vi "Pre-Install Custom Action.vi"(10 "Variant":variant) -> (0 "error out":errorcluster)   [LabVIEW 2020]
uses:
  <resource>/dialog/lvconfig.llb/LV Config Read String.vi
  <resource>/dialog/lvconfig.llb/LV Config Read Numeric (I32).vi
  <vilib>/Utility/config.llb/Write Key (String).vi
  <vilib>/Utility/config.llb/Write Key (I32).vi
  <vilib>/Utility/config.llb/NI_LVConfig.lvlib
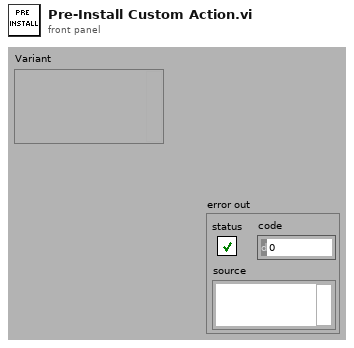
[diagram p1: front panel]
types:
  T1 = typedef "NI_LVConfig.lvlib/Config Data RefNum.ctl" = refnum<k1>
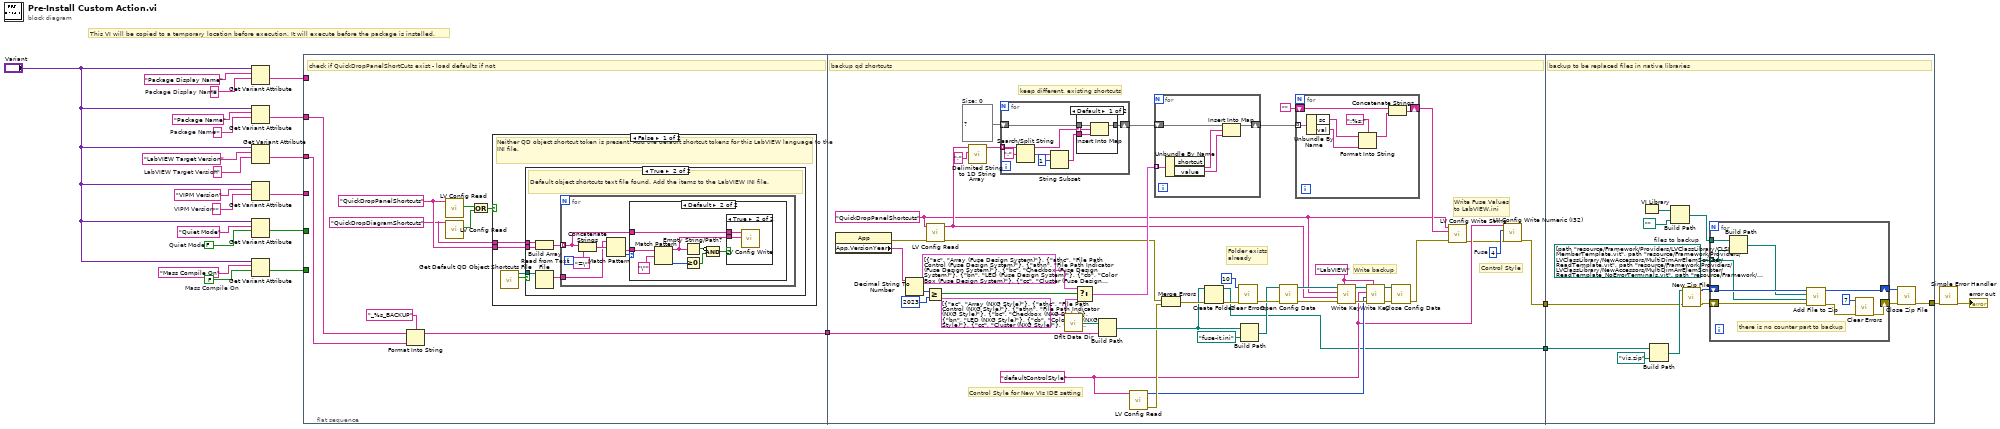
[diagram p0: block diagram]
diagram:
  w6 = FALSE  # Mass Compile On
  w8 = ""  # Package Display Name
  w15 = FALSE  # Quiet Mode
  w18 = ""  # VIPM Version
  w20 = ""  # LabVIEW Target Version
  w22 = ""  # Package Name
  # "This VI will be copied to a temporary location before execution. It will execute before the package is installed."
  n1 = Get Variant Attribute(Variant="Variant", name="Package Display Name", default value (empty Variant)=w8) -> (value=w14:string)  [unwired: 1 in, 3 out]
  n2 = Get Variant Attribute(Variant="Variant", name="Package Name", default value (empty Variant)=w22) -> (value=w13:string)  [unwired: 1 in, 3 out]
  n3 = Get Variant Attribute(Variant="Variant", name="LabVIEW Target Version", default value (empty Variant)=w20) -> (value=w12:string)  [unwired: 1 in, 3 out]
  n4 = Get Variant Attribute(Variant="Variant", name="VIPM Version", default value (empty Variant)=w18) -> (value=w11:string)  [unwired: 1 in, 3 out]
  n5 = Get Variant Attribute(Variant="Variant", name="Quiet Mode", default value (empty Variant)=w15) -> (value=w10:bool)  [unwired: 1 in, 3 out]
  n6 = Get Variant Attribute(Variant="Variant", name="Mass Compile On", default value (empty Variant)=w6) -> (value=w9:bool)  [unwired: 1 in, 3 out]
  n7 = flat-sequence {
    tunnel: w14 -> [_]
    tunnel: w13 -> [w27]
    tunnel: w12 -> [w26]
    tunnel: w11 -> [_]
    tunnel: w10 -> [_]
    tunnel: w9 -> [_]
    tunnel: [w25] -> w4
    tunnel: w4 -> [w85]
    tunnel: [w59] -> w3
    tunnel: [w64] -> w2
    tunnel: [w129] -> w5
    tunnel: w3 -> [w126]
    tunnel: w2 -> [w128]
    frame #0 {
      w32 = "QuickDropDiagramShortcuts" ("Name")
      w33 = "QuickDropPanelShortcuts" ("key")
      # "check if QuickDropPanelShortCuts exist - load defaults if not"
      n8 = Format Into String(format string="_%s_BACKUP", initial string=w27, w26) -> (resulting string=w25:string)  [unwired: 1 in, 1 out]
      n9 = call-poly <resource>:"LV Config Read.vi"("key"=w33) -> ("found?"=w29:bool)  [unwired: 4 in, 2 out]
      n10 = call-poly <resource>:"LV Config Read.vi"("key"=w32) -> ("found?"=w30:bool)  [unwired: 4 in, 2 out]
      n11 = Or(x=w29, y=w30) -> (x .or. y?=w31:bool)
      n12 = case shown="False" w31 {
        tunnel: w32 -> [w37 _]
        tunnel: w33 -> [w36 _]
        frame False {
          # "Neither QD object shortcut token is present. Add the default shortcut tokens for this LabVIEW language to the INI file."
          n13 = call <resource>:"Get Default QD Object Shortcuts File.vi"() -> ("file exists"=w35:bool, "default shortcuts text file"=w34:path)  [unwired: 10 in]
          n14 = case shown="True" w35 {
            tunnel: w34 -> [_ w42]
            tunnel: w37 -> [_ w40]
            tunnel: w36 -> [_ w39]
            frame False {
              # "Default object shortcuts text file does not exist for this language. Do nothing."
            }
            frame True {
              # "Default object shortcuts text file found. Add the items to the LabVIEW INI file."
              n15 = Build Array(w40, w39) -> (w38:string[])
              n16 = Read from Text File(file (use dialog)=w42) -> (text=w41:string)  [unwired: 3 in, 3 out]
              n17 = for {
                tunnel: w41 -> [w44]
                tunnel: w38 -> [w46] mode=indexing
                n18 = Concatenate Strings(w46, "=\"") -> (w45:string)
                n19 = Match Pattern(string=w44, regular expression=w45) -> (after substring=w47:string, offset past match=w43:i32)  [unwired: 1 in, 2 out]
                n20 = case shown="Default" w43 {
                  tunnel: w47 -> [_ w56]
                  tunnel: w46 -> [_ w54]
                  frame -1 {
                  }
                  frame Default {
                    n21 = Match Pattern(string=w56, regular expression="\"") -> (before substring=w53:string, offset past match=w51:i32)  [unwired: 1 in, 2 out]
                    n22 = Empty String/Path?(string/path=w53) -> (empty?=w52:bool)
                    n23 = Greater Or Equal To 0?(x=w51) -> (x >= 0?=w50:bool)
                    n24 = Compound Arithmetic op=AND(invert w52, w50) -> (w49:bool)
                    n25 = case shown="True" w49 {
                      tunnel: w54 -> [_ w58]
                      tunnel: w53 -> [_ w57]
                      frame False {
                      }
                      frame True {
                        n26 = call-poly <resource>:"LV Config Write.vi"("value"=w57, "key"=w58) -> ()  [unwired: 5 in, 1 out]
                      }
                    }
                  }
                }
              }
            }
          }
        }
        frame True {
          # "One or both of the QD object shortcut tokens is already present, don't do anything with loading default shortcuts."
        }
      }
    }
    frame #1 {
      w62 = u32 4  # Fuse
      w63 = "defaultControlStyle" ("key")
      w98 = map{string, string} {}  # Size: 0
      w60 = "QuickDropPanelShortcuts" ("key")
      w72 = "LabVIEW" ("section")
      # "Write backup"
      # "Write Fuse Values\nto LabVIEW.ini"
      # "keep different, existing shortcuts"
      # "Control Style"
      # "Control Style for New VIs IDE setting"
      # "Folder exists\nalready"
      # "backup qd shortcuts"
      n27 = property class="App"() -> (error out=w71:errorcluster, "App.VersionYear"=w91:string)  [unwired: 2 in, 1 out]
      n28 = Decimal String To Number(string=w91) -> (number=w90:i32)  [unwired: 2 in, 1 out]
      n29 = Greater Or Equal?(x=w90, y=2023) -> (x >= y?=w88:bool)
      n30 = call-poly <resource>:"LV Config Read.vi"("error in"=w71, "key"=w60) -> ("error out"=w70:errorcluster, "value"=w69:string)  [unwired: 3 in, 1 out]
      n31 = call <vilib>:"Delimited String to 1D String Array.vi"("delimiter"=";", "delimited string"=w69) -> ("string array"=w99:string[])  [unwired: 9 in]
      n32 = for {
        tunnel: w99 -> [w119] mode=indexing
        shift-right: [w117] -> w97
        shift-left: w98 -> [w118]
        n33 = Search/Split String(string=w119, search string/char (-)=":") -> (substring before match=w116:string, match + rest of string=w115:string)  [unwired: 1 in, 1 out]
        n34 = String Subset(string=w115, offset (0)=1) -> (substring=w114:string)  [unwired: 1 in]
        n35 = case shown="Default" w116 {
          selector: w116 -> [w122 _]
          tunnel: w118 -> [w124 w125]
          tunnel: [w123 w125] -> w117
          tunnel: w114 -> [w121 _]
          frame Default {
            n36 = Insert Into Map(map in=w124, key=w122, value=w121) -> (map out=w123:map{string, string})  [unwired: 2 out]
          }
          frame "" {
          }
        }
      }
      n37 = call <vilib>:"Dflt Data Dir.vi"() -> ("App:Default Data Directory"=w87:path)
      n38 = Select(t=cluster{"shortcut":string, "value":string}[] [{"shortcut"="ac", "value"="Array (Fuse Design System)"}, {"shortcut"="athc", "value"="File Path Control (Fuse Design System)"}, {"shortcut"="athn", "value"="File Path Indicator (Fuse Design System)"}, {"shortcut"="bc", "value"="Checkbox (Fuse Design System)"}, {"shortcut"="bn", "value"="LED (Fuse Design System)"}, {"shortcut"="cb", "value"="Color Box (Fuse Design System)"}, {"shortcut"="cc", "value"="Cluster (Fuse Design System)"}, {"shortcut"="cr", "value"="Control Refnum"}, {"shortcut"="en", "value"="Enum (Fuse Design System)"}, {"shortcut"="erc", "value"="Error In  (Fuse Design System)"}, {"shortcut"="ern", "value"="Error Out (Fuse Design System)"}, {"shortcut"="nc", "value"="Numeric Control (Fuse Design System)"}, {"shortcut"="nn", "value"="Numeric Indicator (Fuse Design System)"}, {"shortcut"="sac", "value"="Select a Control..."}, {"shortcut"="sc", "value"="String Control (Fuse Design System)"}, {"shortcut"="sn", "value"="String Indicator (Fuse Design System)"}, {"shortcut"="vr", "value"="VI Refnum"}, {"shortcut"="wc", "value"="Waveform Chart (Fuse Design System)"}, {"shortcut"="wg", "value"="Waveform Graph (Fuse Design System)"}, {"shortcut"="xg", "value"="XY Graph (Fuse Design System)"}] ("Array"), s=w88, f=cluster{"shortcut":string, "value":string}[] [{"shortcut"="ac", "value"="Array (NXG Style)"}, {"shortcut"="athc", "value"="File Path Control (NXG Style)"}, {"shortcut"="athn", "value"="File Path Indicator (NXG Style)"}, {"shortcut"="bc", "value"="Checkbox (NXG Style)"}, {"shortcut"="bn", "value"="LED (NXG Style)"}, {"shortcut"="cb", "value"="Color Box (NXG Style)"}, {"shortcut"="cc", "value"="Cluster (NXG Style)"}, {"shortcut"="cr", "value"="Control Refnum"}, {"shortcut"="en", "value"="Enum (NXG Style)"}, {"shortcut"="erc", "value"="Error In  (NXG Style)"}, {"shortcut"="ern", "value"="Error Out (NXG Style)"}, {"shortcut"="nc", "value"="Numeric Control (NXG Style)"}, {"shortcut"="nn", "value"="Numeric Indicator (NXG Style)"}, {"shortcut"="sac", "value"="Select a Control..."}, {"shortcut"="sc", "value"="String Control (NXG Style)"}, {"shortcut"="sn", "value"="String Indicator (NXG Style)"}, {"shortcut"="vr", "value"="VI Refnum"}, {"shortcut"="wc", "value"="Waveform Chart (NXG Style)"}, {"shortcut"="wg", "value"="Waveform Graph (NXG Style)"}, {"shortcut"="xg", "value"="XY Graph (NXG Style)"}] ("Array")) -> (s? t:f=w93:cluster{"shortcut":string, "value":string}[])
      n39 = Build Path(base path=w87, name or relative path=w85) -> (appended path=w73:path)
      n40 = call-poly <resource>:"LV Config Read.vi"("key"=w63) -> ("error out"=w68:errorcluster, "value"=w67:i32)  [unwired: 4 in, 1 out]
      n41 = for {
        tunnel: w93 -> [w110] mode=indexing
        shift-right: [w111] -> w96
        shift-left: w97 -> [w112]
        n42 = Unbundle By Name(w110) -> ("shortcut"=w109:string, "value"=w108:string)
        n43 = Insert Into Map(map in=w112, key=w109, value=w108) -> (map out=w111:map{string, string})  [unwired: 2 out]
      }
      n44 = Merge Errors(w70, w68) -> (w74:errorcluster)
      n45 = Create Folder(path (use dialog)=w73, error in=w74) -> (created path=w59:path, error out=w75:errorcluster)  [unwired: 1 in, 1 out]
      n46 = call <vilib>:"Clear Errors.vi"("error in (no error)"=w75, "specific error code to clear (0: all)"=10) -> ("error out"=w84:errorcluster)  [unwired: 4 in, 1 out]
      n47 = Build Path(base path=w73, name or relative path=path "fuse-it.ini") -> (appended path=w76:path)
      n48 = call <vilib>:"Open Config Data.vi"("error in (no error)"=w84, "configuration file path"=w76) -> ("error out"=w82:errorcluster, "refnum"=w81:T1)  [unwired: 7 in, 1 out]
      n49 = for {
        tunnel: w96 -> [w107] mode=indexing
        shift-right: [w103] -> w65
        shift-left: "" -> [w105]
        n50 = Unbundle By Name(w107) -> ("sc"=w101:string, "val"=w102:string)
        n51 = Format Into String(format string=":%s;", initial string=w101, w102) -> (resulting string=w104:string)  [unwired: 1 in, 1 out]
        n52 = Concatenate Strings(w105, w104) -> (w103:string)
      }
      n53 = call-poly <vilib>:"Write Key.vi"("section"=w72, "error in (no error)"=w82, "value"=w69, "key"=w60, "refnum"=w81) -> ("error out"=w80:errorcluster, "refnum out"=w79:T1)  [unwired: 4 in, 1 out]
      n54 = call-poly <vilib>:"Write Key.vi"("section"=w72, "error in (no error)"=w80, "value"=w67, "key"=w63, "refnum"=w79) -> ("error out"=w78:errorcluster, "refnum out"=w77:T1)  [unwired: 4 in, 1 out]
      n55 = call <vilib>:"Close Config Data.vi"("error in (no error)"=w78, "refnum"=w77) -> ("error out"=w66:errorcluster)  [unwired: 8 in, 1 out]
      n56 = call <resource>:"LV Config Write String.vi"("error in (no error)"=w66, "value"=w65, "key"=w60) -> ("error out"=w61:errorcluster)  [unwired: 4 in]
      n57 = call <resource>:"LV Config Write Numeric (I32).vi"("error in (no error)"=w61, "value"=w62, "key"=w63) -> ("error out"=w64:errorcluster)  [unwired: 4 in]
    }
    frame #2 {
      w127 = path[] [path "resource/Framework/Providers/LVClassLibrary/CLSUIP_MemberTemplate.vit", path "resource/Framework/Providers/LVClassLibrary/NewAccessors/MultiDimArrElemScripter/ReadTemplate.vit", path "resource/Framework/Providers/LVClassLibrary/NewAccessors/MultiDimArrElemScripter/ReadTemplate_NoErrorTerminals.vit", path "resource/Framework/Providers/LVClassLibrary/NewAccessors/MultiDimArrElemScripter/WriteTemplate.vit", path "resource/Framework/Providers/LVClassLibrary/NewAccessors/MultiDimArrElemScripter/WriteTemplate_NoErrorTerminals.vit", path "resource/Framework/Providers/LVClassLibrary/NewAccessors/BaseAccessorScripter/ReadTemplate.vit", path "resource/Framework/Providers/LVClassLibrary/NewAccessors/BaseAccessorScripter/ReadTemplate_NoErrorTerminals.vit", path "resource/Framework/Providers/LVClassLibrary/NewAccessors/BaseAccessorScripter/WriteTemplate.vit", path "resource/Framework/Providers/LVClassLibrary/NewAccessors/BaseAccessorScripter/WriteTemplate_NoErrorTerminals.vit", path "resource/Framework/Providers/LVClassLibrary/NewAccessors/ArrayElementScripter/ReadTemplate.vit", path "resource/Framework/Providers/LVClassLibrary/NewAccessors/ArrayElementScripter/ReadTemplate_NoErrorTerminals.vit", path "resource/Framework/Providers/LVClassLibrary/NewAccessors/ArrayElementScripter/WriteTemplate.vit", path "resource/Framework/Providers/LVClassLibrary/NewAccessors/ArrayElementScripter/WriteTemplate_NoErrorTerminals.vit"]  # files to backup
      # "backup to be replaced files in native libraries"
      n58 = VI Library() -> (path=w134:path)
      n59 = Build Path(base path=w126, name or relative path=path "vis.zip") -> (appended path=w130:path)
      n60 = Build Path(base path=w134, name or relative path=path "..") -> (appended path=w132:path)
      n61 = call <vilib>:"New Zip File.vi"("error in (no error)"=w128, "target"=w130) -> ("error out"=w137:errorcluster, "zip file out"=w138:i64)  [unwired: 3 in, 1 out]
      n62 = for {
        tunnel: w127 -> [w139] mode=indexing
        shift-right: [w142] -> w136
        shift-left: w137 -> [w144]
        shift-right: [w145] -> w135
        shift-left: w138 -> [w146]
        tunnel: w132 -> [w140]
        # "there is no counter part to backup"
        n63 = Build Path(base path=w140, name or relative path=w139) -> (appended path=w143:path)
        n64 = call <vilib>:"Add File to Zip.vi"("error in (no error)"=w144, "destination path in zip"=w139, "source file path"=w143, "zip file in"=w146) -> ("error out"=w147:errorcluster, "zip file out"=w145:i64)  [unwired: 6 in]
        n65 = call <vilib>:"Clear Errors.vi"("error in (no error)"=w147, "specific error code to clear (0: all)"=7) -> ("error out"=w142:errorcluster)  [unwired: 4 in, 1 out]
      }
      n66 = call <vilib>:"Close Zip File.vi"("error in (no error)"=w136, "zip file in"=w135) -> ("error out"=w129:errorcluster)  [unwired: 5 in]
    }
  }
  n67 = call <vilib>:"Simple Error Handler.vi"("error in (no error)"=w5) -> ("error out"=→"error out":errorcluster)  [unwired: 4 in, 4 out]
